vi "SMTP Email Send File Attachment.vi"(5 "translit":string, 6 "binary? (F)":bool, 7 "character set":string, 8 "error in (no error)":errorcluster, 10 "path":path, 11 "smtp session":T1) -> (0 "error out":errorcluster, 2 "file error":errorcluster, 3 "smtp session out":T1)   [LabVIEW 2009, in "NewNI_SMTPEmail.lvlib"]
doc: "Writes the file specified by the \"refnum\" into TCP connection specified by \"connection ID\". In case the file is a text file the appropriate conversions are performed, where 8-bit characters (ASCII values over 127) are encoded using quoted-printable encoding. In case the file is binary, base64 encoding is used.\n\nFile Type: Type of file, can be either text or binary. By default it is text (corresponds to True). False means binary.\n\nFile Size: Size of the file in bytes."
uses:
  NewNI_SMTPEmail.lvlib
  SMTP Email Session.ctl
panel:
  in  "buffered tcp connection":refnum<k5>
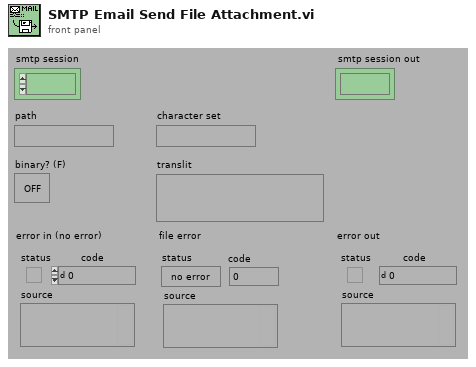
[diagram p1: front panel]
types:
  T1 = typedef "NewNI_SMTPEmail.lvlib/SMTP Email Session.ctl" = refnum<k1>
  T2 = enum16{"read/write", "read-only", "write-only", "write-only (truncate)"}
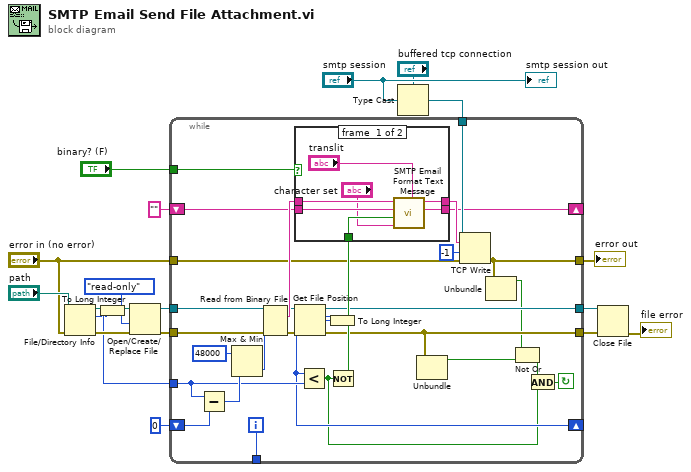
[diagram p0: block diagram]
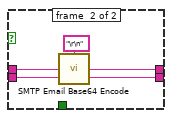
[diagram p2: hidden frame]
diagram:
  n1 = File/Directory Info(path="path", error in="error in (no error)") -> (path out=w15:path, size=w1:i64, error out=w11:errorcluster)  [unwired: 4 out]
  n2 = To Long Integer(number=w1) -> (32bit integer=w9:i32)
  n3 = Open/Create/Replace File(file path (use dialog)=w15, error in=w11, access (0:read/write)=T2."read-only" ("open mode (0)")) -> (refnum out=w13:refnum<file>, error out=w14:errorcluster)  [unwired: 4 out]
  n4 = Type Cast(type="buffered tcp connection", x="smtp session") -> (*(type *) &x=w2:refnum<k5>)
  n5 = while {
    tunnel: [w25] -> _
    tunnel: [w31] -> w6
    tunnel: [w32] -> w7
    tunnel: "error in (no error)" -> [w33]
    shift-left: "" ("next data") -> [w37]
    shift-right: [w36] -> _
    tunnel: "binary? (F)" -> [w40]
    tunnel: w13 -> [w41]
    tunnel: w2 -> [w42]
    tunnel: [w34] -> w19
    tunnel: w9 -> [w28]
    tunnel: w14 -> [w48]
    shift-left: 0 ("offset") -> [w27]
    shift-right: [w26] -> _
    i -> [w25]
    stop <- w43 continue-if-true
    n6 = Subtract(x=w28, y=w27) -> (x-y=w45:i32)
    n7 = Max & Min(x=48000, y=w45) -> (min(x,y)=w47:i32)  [unwired: 1 out]
    n8 = Read from Binary File(8:w48, 10:w47, 11:w41) -> (0:w21:errorcluster, 2:w39:string, 3:w22:refnum<file>)  [unwired: 4 out]
    n9 = Get File Position(4:w21, 7:w22) -> (0:w31:errorcluster, 2:w20:i64, 3:w32:refnum<file>)
    n10 = To Long Integer(number=w20) -> (32bit integer=w26:i32)
    n11 = Less?(x=w26, y=w28) -> (x < y?=w23:bool)
    n12 = Not(x=w23) -> (.not. x?=w35:bool)
    n13 = case shown="False" w40 {
      tunnel: w39 -> [w55 w58]
      tunnel: [w54 w57] -> w38
      tunnel: w37 -> [w53 w56]
      tunnel: [w52 w56] -> w36
      tunnel: w35 -> [w51 _]
      frame #0 {
        n14 = call "SMTP Email Format Text Message.vi"("translit"="translit", "character set"="character set", "last chunk (T)"=w51, "prev data (\"\")"=w53, "text"=w55) -> ("next data"=w52:string, "formated text"=w54:string)  [unwired: 3 out]
      }
      frame #1 {
        n15 = call "SMTP Email Base64 Encode.vi"("Normal String"=w58, "Line separator (\\n)"="\r\n") -> ("Base64 String"=w57:string)
      }
    }
    n16 = Unbundle(w31) -> ("status"=w29:bool)  [unwired: 2 out]
    n17 = TCP Write(connection ID=w42, data in=w38, error in (no error)=w33, 9:-1 ("timeout ms (25000)")) -> (error out=w34:errorcluster)  [unwired: 2 out]
    n18 = Unbundle(w34) -> ("status"=w30:bool)  [unwired: 2 out]
    n19 = Not Or(1:w29, 2:w30) -> (0:w44:bool)
    n20 = And(x=w44, y=w23) -> (x .and. y?=w43:bool)
  }
  "error out" <- w19
  n21 = Close File(refnum=w7, error in=w6) -> (error out=→"file error":errorcluster)  [unwired: 1 out]
  "smtp session out" <- "smtp session"
